vi "DIE.vi"() -> ()   [LabVIEW 2012]
uses:
  <instrlib>/niScope/Controls/niScope trigger source.ctl
  <instrlib>/niScope/Controls/niScope vertical coupling.ctl
  <instrlib>/niScope/Configure/Trigger/niScope Configure Trigger Edge.vi
  <instrlib>/niScope/Acquire/Fetch/niScope Multi Fetch Cluster.vi
panel:
  in  "Signal Coupling":T1=1 caption="vertical coupling" items=["AC", "DC", "Ground"]
  in  "Signal Source":T2="1"
  in  "Reference Position (%)":dbl=50.0 caption="Reference Position" format="%.1f"
  out "Total Acquisition Time (s)":dbl
  out "Scope Traces":dbl[](graph)
  in  "min sample rate":dbl=1000000.0 caption="Sample Rate (Max 20M)" format="%^.2e"
  in  "Trigger Level":dbl=2.0 format="%.2f"
  in  "Trigger Source":T2="0"
  in  "Number of Records":i32=1000 caption="Number of Samples"
  # "Settings can be modified \nin real-time (every 10s or so)."
  # "For smooth sailing, keep this value below 9s."
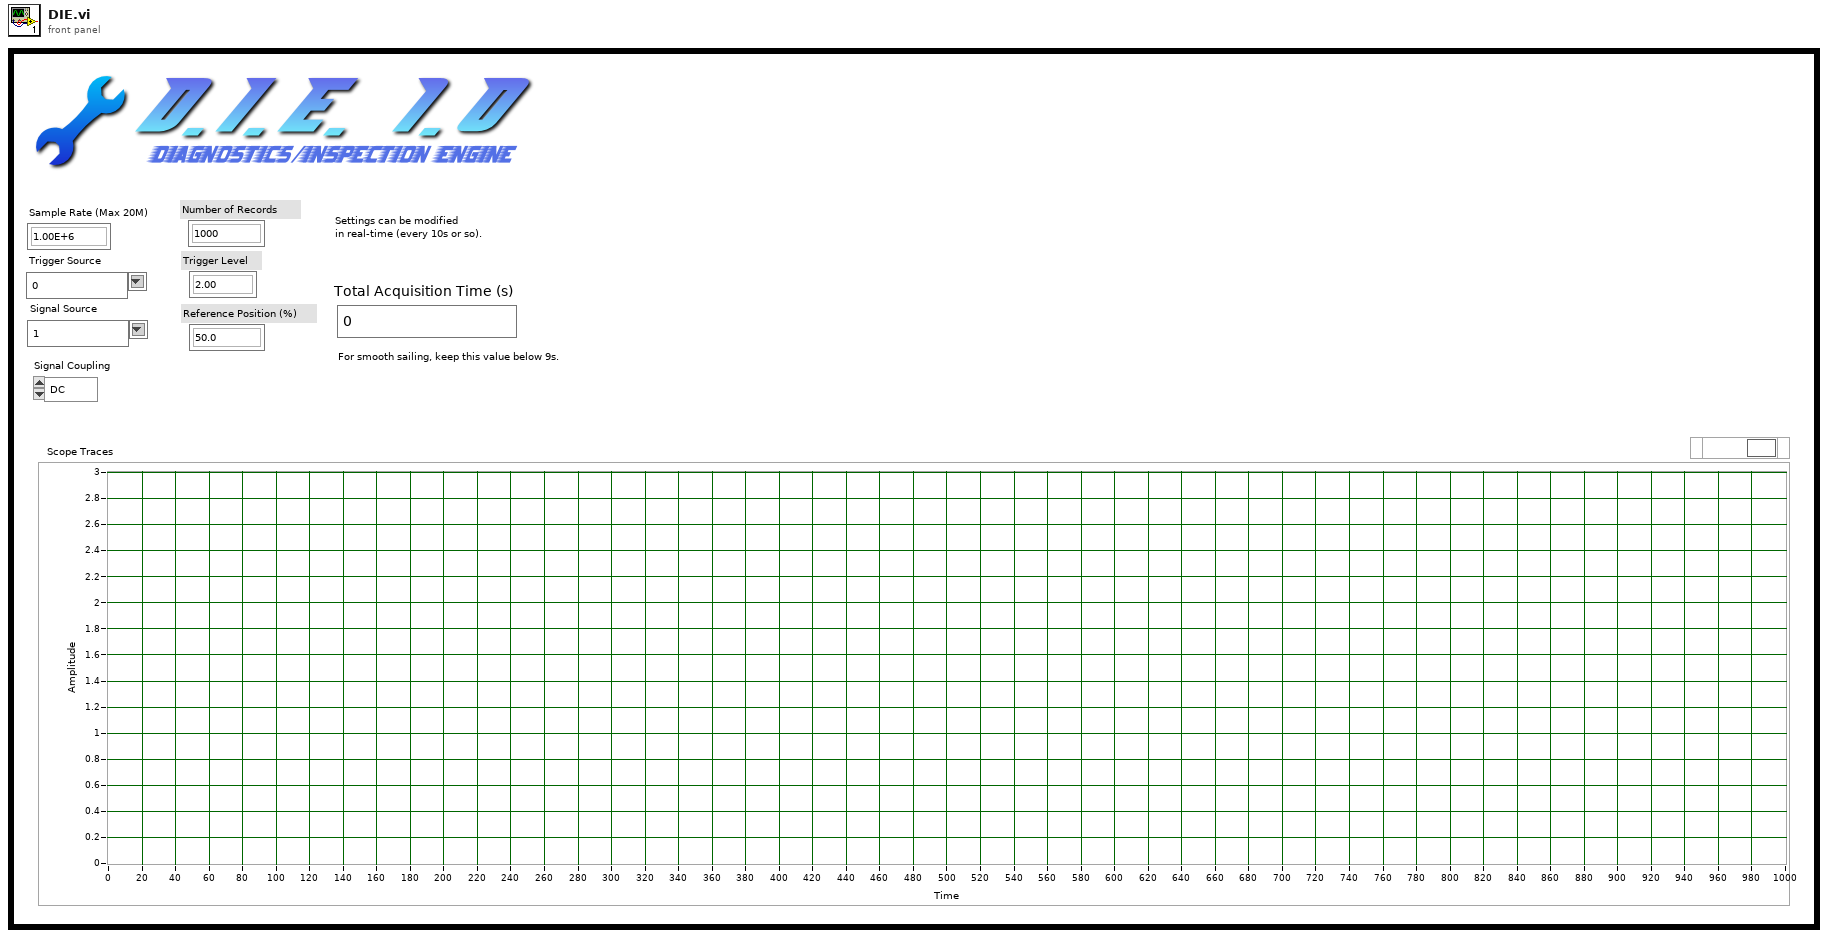
[diagram p1: front panel]
types:
  T1 = typedef "niScope vertical coupling.ctl" = i32
  T2 = typedef "niScope trigger source.ctl" = string
  T3 = cluster{"relativeInitialX":dbl, "xIncrement":dbl, "wfm":dbl[]}[]
  T4 = cluster{"relativeInitialX":dbl, "xIncrement":dbl, "wfm":dbl[]}
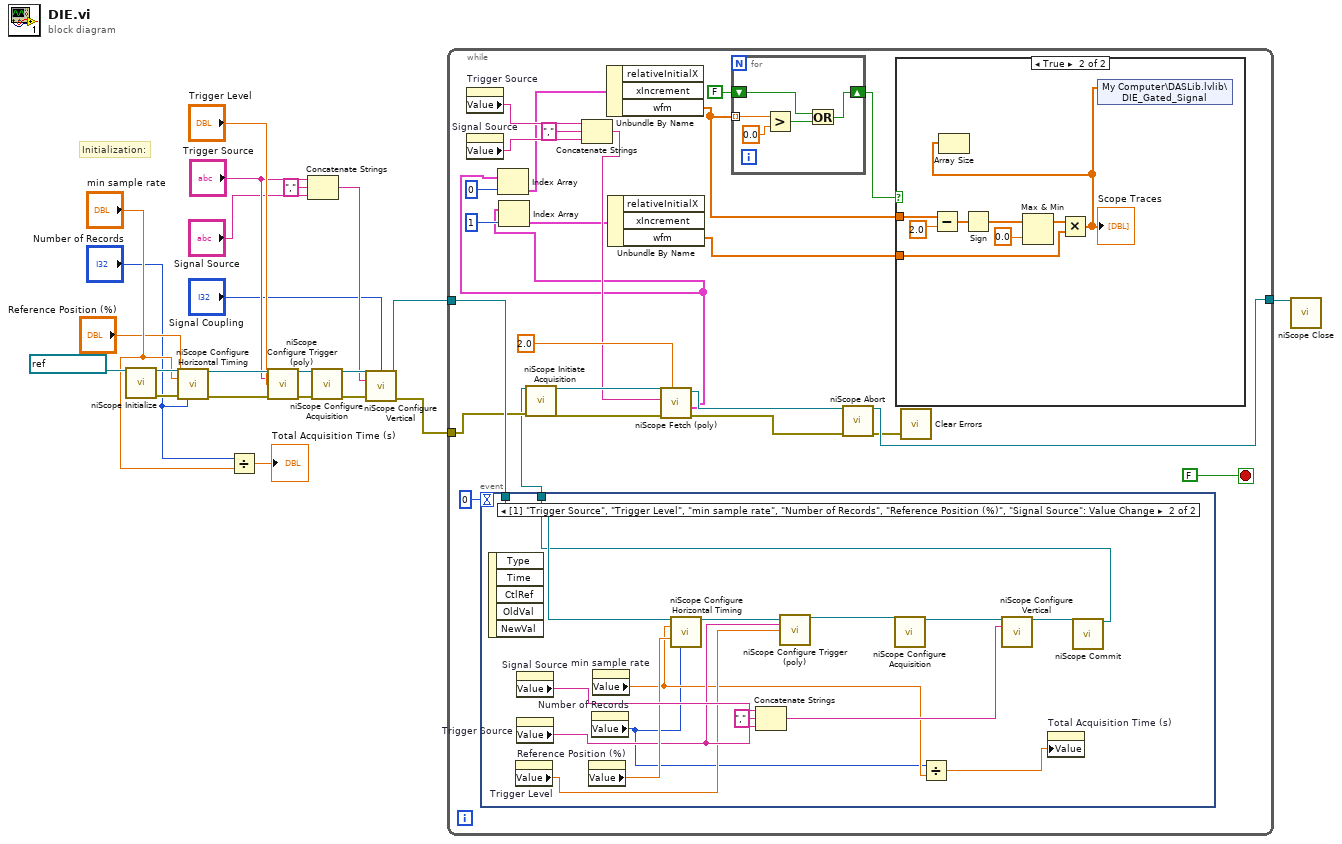
[diagram p0: block diagram]
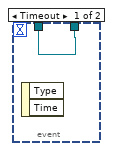
[diagram p2: hidden frame]
diagram:
  # "Initialization:"
  n1 = call <instrlib>:"niScope Initialize.vi"("resource name"=refnum<k15> "PXI1Slot4") -> ("instrument handle"=w21:refnum<k15>, "error out"=w20:errorcluster)  [unwired: 13 in]
  n2 = call <instrlib>:"niScope Configure Horizontal Timing.vi"("instrument handle"=w21, "min sample rate"="min sample rate", "reference position"="Reference Position (%)", "error in"=w20, "min record length"="Number of Records") -> ("instrument handle out"=w19:refnum<k15>, "error out"=w10:errorcluster)  [unwired: 9 in]
  n3 = Divide(x="Number of Records", y="min sample rate") -> (x/y=→"Total Acquisition Time (s)":dbl)
  n4 = call-poly <instrlib>:"niScope Configure Trigger (poly).vi"("instrument handle"=w19, "trigger source"="Trigger Source", "trigger level"="Trigger Level", "error in"=w10) -> ("instrument handle out"=w16:refnum<k15>, "error out"=w15:errorcluster)  [unwired: 10 in]
  n5 = Concatenate Strings("Trigger Source", "," ("string"), "Signal Source") -> (w3:string)
  n6 = call <instrlib>:"niScope Configure Acquisition.vi"("instrument handle"=w16, "error in"=w15) -> ("instrument handle out"=w13:refnum<k15>, "error out"=w14:errorcluster)  [unwired: 12 in]
  n7 = call <instrlib>:"niScope Configure Vertical.vi"("instrument handle"=w13, "vertical coupling"="Signal Coupling", "channels"=w3, "error in"=w14) -> ("instrument handle out"=w17:refnum<k15>, "error out"=w12:errorcluster)  [unwired: 10 in]
  n8 = while {
    tunnel: w17 -> [w37]
    tunnel: w12 -> [w36]
    tunnel: [w46] -> w11
    stop <- FALSE ("stop") stop-if-true
    n9 = property on="Trigger Source" class="CmbBox (strict)"() -> ("Value"=w33:T2)  [unwired: 2 in, 2 out]
    n10 = property on="Signal Source" class="CmbBox (strict)"() -> ("Value"=w31:T2)  [unwired: 2 in, 2 out]
    n11 = event shown="[1] \"Trigger Source\", \"Trigger Level\", \"min sample rate\", \"Number of Records\", \"Reference Position (%)\", \"Signal Source\": Value Change" {
      selector: _ -> [_ _]
      dyn-events: _ -> [_ _]
      timeout: 0 -> [_ _]
      tunnel: w37 -> [w48 w63]
      tunnel: [w48 w50] -> w23
      event Timeout {
        n12 = event-data() -> ()  [unwired: 1 in, 2 out]
      }
      event "Trigger Level", "min sample rate", "Number of Records", "Reference Position (%)": Value Change {
        n13 = event-data() -> ()  [unwired: 1 in, 5 out]
        n14 = property on="Trigger Level" class="DigNum (strict)"() -> ("Value"=w54:dbl)  [unwired: 2 in, 2 out]
        n15 = property on="Signal Source" class="CmbBox (strict)"() -> ("Value"=w57:T2)  [unwired: 2 in, 2 out]
        n16 = property on="Trigger Source" class="CmbBox (strict)"() -> ("Value"=w55:T2)  [unwired: 2 in, 2 out]
        n17 = property on="Reference Position (%)" class="DigNum (strict)"() -> ("Value"=w56:dbl)  [unwired: 2 in, 2 out]
        n18 = property on="Number of Records" class="DigNum (strict)"() -> ("Value"=w49:i32)  [unwired: 2 in, 2 out]
        n19 = property on="min sample rate" class="DigNum (strict)"() -> ("Value"=w53:dbl)  [unwired: 2 in, 2 out]
        n20 = call <instrlib>:"niScope Configure Horizontal Timing.vi"("instrument handle"=w63, "min sample rate"=w53, "reference position"=w56, "min record length"=w49) -> ("instrument handle out"=w62:refnum<k15>)  [unwired: 10 in, 1 out]
        n21 = Concatenate Strings(w57, "," ("string"), w55) -> (w59:string)
        n22 = call-poly <instrlib>:"niScope Configure Trigger (poly).vi"("instrument handle"=w62, "trigger source"=w55, "trigger level"=w54) -> ("instrument handle out"=w61:refnum<k15>)  [unwired: 11 in, 1 out]
        n23 = call <instrlib>:"niScope Configure Acquisition.vi"("instrument handle"=w61) -> ("instrument handle out"=w60:refnum<k15>)  [unwired: 13 in, 1 out]
        n24 = Divide(x=w49, y=w53) -> (x/y=w52:dbl)
        n25 = call <instrlib>:"niScope Configure Vertical.vi"("instrument handle"=w60, "channels"=w59) -> ("instrument handle out"=w51:refnum<k15>)  [unwired: 12 in, 1 out]
        n26 = property on="Total Acquisition Time (s)" class="DigNum (strict)"("Value"=w52) -> ()  [unwired: 2 in, 2 out]
        n27 = call <instrlib>:"niScope Commit.vi"("instrument handle"=w51) -> ("instrument handle out"=w50:refnum<k15>)  [unwired: 13 in, 1 out]
      }
    }
    n28 = call <instrlib>:"niScope Initiate Acquisition.vi"("instrument handle"=w23, "error in"=w36) -> ("instrument handle out"=w35:refnum<k15>, "error out"=w29:errorcluster)  [unwired: 12 in]
    n29 = Concatenate Strings(w33, "," ("string"), w31) -> (w30:string)
    n30 = call-poly <instrlib>:"niScope Fetch (poly).vi"("timeout"=2.0, "error in"=w29, "channels"=w30, "instrument handle"=w35) -> ("error out"=w28:errorcluster, "waveform"=w26:T3, "instrument handle out"=w27:refnum<k15>)  [unwired: 4 in, 1 out]
    n31 = Index Array(array=w26, index=0) -> (element=w25:T4)
    n32 = Index Array(array=w26, index=1) -> (element=w24:T4)
    n33 = Unbundle By Name(w25) -> ("wfm"=w41:dbl[])  [unwired: 2 out]
    n34 = Unbundle By Name(w24) -> ("wfm"=w39:dbl[])  [unwired: 2 out]
    n35 = for {
      tunnel: w41 -> [w64] mode=indexing
      shift-right: [w65] -> w42
      shift-left: FALSE -> [w66]
      n36 = Greater?(x=w64, y=0.0) -> (0:w67:bool)
      n37 = Or(x=w66, y=w67) -> (x .or. y?=w65:bool)
    }
    n38 = call <instrlib>:"niScope Abort.vi"("instrument handle"=w27, "error in"=w28) -> ("instrument handle out"=w46:refnum<k15>, "error out"=w45:errorcluster)  [unwired: 12 in]
    n39 = case shown="True" w42 {
      tunnel: w41 -> [_ w71]
      tunnel: w39 -> [_ w70]
      frame False {
      }
      frame True {
        n40 = Subtract(x=w71, y=2.0 ("timeout")) -> (x-y=w75:dbl[])
        n41 = Sign(1:w75) -> (0:w74:dbl[])
        n42 = Max & Min(x=w74, y=0.0 ("timeout")) -> (max(x,y)=w72:dbl[])  [unwired: 1 out]
        n43 = Multiply(x=w72, y=w70) -> (x*y=w69:dbl[])
        "Scope Traces" <- w69
        n44 = Array Size(array=w69) -> ()  [unwired: 1 out]
        n45 = shared-variable "My Computer\\DASLib.lvlib\\DIE_Gated_Signal"(w69) -> ()  [unwired: 1 in, 1 out]
      }
    }
    n46 = call <vilib>:"Clear Errors.vi"("error in (no error)"=w45) -> ()  [unwired: 6 in, 1 out]
  }
  n47 = call <instrlib>:"niScope Close.vi"("instrument handle"=w11) -> ()  [unwired: 14 in, 1 out]
